vi "exo4.vi"() -> ()   [LabVIEW 2019]
uses:
  <vilib>/myRIO/Instrument Drivers/Onboard IO/I2C/typedefs/I2C User Configuration.ctl
  <vilib>/myRIO/Instrument Drivers/Onboard IO/I2C/typedefs/I2C Transfer Rate.ctl
  <vilib>/myRIO/Instrument Drivers/Onboard IO/I2C/typedefs/I2C Reference.ctl
  <vilib>/myRIO/Common/Instrument Driver Framework/Utilities/typedefs/myRIO Generic Hardware Reference.ctl
  <vilib>/myRIO/Common/Instrument Driver Framework/Utilities/typedefs/Hardware Version Enum.ctl
  <vilib>/myRIO/Common/Instrument Driver Framework/Utilities/typedefs/myRIO v1.0 Reference.ctl
  <vilib>/myRIO/Common/Instrument Driver Framework/Utilities/typedefs/Generic FPGA Reference.ctl
  <vilib>/myRIO/Common/Instrument Driver Framework/myRIO v1.0/I2C/typedefs/I2C Channels Enum.ctl
  <vilib>/myRIO/Instrument Drivers/Onboard IO/I2C/typedefs/I2C Configuration.ctl
  <vilib>/userDefined/High Color/nirio_resource_hc.ctl
  <vilib>/myRIO/Common/Instrument Driver Framework/Utilities/vis/Is FPGA Ref Available.vi
  <vilib>/myRIO/Common/Instrument Driver Framework/myRIO v1.0/I2C/vis/myRIO v1.1 Open I2C.vi
  <vilib>/myRIO/Instrument Drivers/Onboard IO/I2C/vis/Configure.vi
  <vilib>/myRIO/Instrument Drivers/Onboard IO/I2C/vis/Write.vi
  <vilib>/myRIO/Instrument Drivers/Onboard IO/I2C/vis/Read.vi
  <vilib>/myRIO/Common/Instrument Driver Framework/Utilities/vis/Validate Channels.vi
  <vilib>/myRIO/Common/Instrument Driver Framework/myRIO v1.0/I2C/vis/myRIO v1.0 Reserve I2C.vi
  <vilib>/myRIO/Common/Instrument Driver Framework/myRIO v1.0/I2C/vis/myRIO v1.0 Build MUX Configuration I2C.vi
  <vilib>/myRIO/Common/Instrument Driver Framework/myRIO v1.0/Resource Manager/vis/myRIO v1.0 Reserve Channel List.vi
  <vilib>/myRIO/Common/Instrument Driver Framework/myRIO v1.0/Resource Manager/vis/myRIO v1.0 Create Configuration List.vi
  <vilib>/myRIO/Common/Instrument Driver Framework/myRIO v1.0/Resource Manager/vis/myRIO v1.0 Reserve Channel.vi
  <vilib>/myRIO/Common/Instrument Driver Framework/myRIO v1.0/Resource Manager/vis/myRIO v1.0 Unreserve Channel.vi
  <vilib>/myRIO/Common/Instrument Driver Framework/myRIO v1.0/Resource Manager/vis/myRIO v1.0 Build Mutex Name.vi
  <vilib>/Utility/VariantDataType/GetNumericInfo.vi
  <vilib>/Utility/error.llb/Error Cluster From Error Code.vi
  <vilib>/myRIO/Common/Instrument Driver Framework/myRIO v1.0/myRIO v1.1 Open.vi
  <vilib>/myRIO/Common/Instrument Driver Framework/Utilities/vis/IO Manager.vi
  <vilib>/myRIO/Common/Instrument Driver Framework/Utilities/vis/Configuration Manager.vi
  <vilib>/myRIO/Common/Instrument Driver Framework/myRIO v1.0/Resource Manager/vis/myRIO v1.0 Configure IO.vi
  <vilib>/myRIO/Common/Instrument Driver Framework/myRIO v1.0/myRIO v1.0 Close.vi
  <vilib>/myRIO/Common/Instrument Driver Framework/myRIO v1.0/I2C/vis/myRIO v1.0 Configure I2C.vi
  <vilib>/myRIO/Common/Instrument Driver Framework/myRIO v1.0/I2C/vis/myRIO v1.0 Write I2C.vi
  <vilib>/myRIO/Common/Instrument Driver Framework/myRIO v1.0/I2C/vis/myRIO v1.0 Read I2C.vi
  <vilib>/myRIO/Express VI/Onboard IO/I2C/I2C Express VI.xnode
  <vilib>/myRIO/Instrument Drivers/Onboard IO/I2C/vis/myRIO I2C Open.xnode
  <vilib>/myRIO/Instrument Drivers/Onboard IO/I2C/I2C.lvlib
panel:
  out "Bytes Read Z high magnetometer":u8[](array[numeric])
  out "Bytes Read Y high magnetometer":u8[](array[numeric])
  out "Bytes Read X high magnetometer":u8[](array[numeric])
  out "Bytes Bytes Read Z low magnetometer":u8[](array[numeric])
  out "Bytes Bytes Read Y low magnetometer":u8[](array[numeric])
  out "Bytes Bytes Read X low magnetometer":u8[](array[numeric])
  out "Bytes Read Z high accelerometer":u8[](array[numeric])
  out "Bytes Read Y high accelerometer":u8[](array[numeric])
  out "Bytes Read X high accelerometer":u8[](array[numeric])
  out "Bytes Read Z low accelerometer":u8[](array[numeric])
  out "Bytes Read Y low accelerometer":u8[](array[numeric])
  out "Bytes Read X low accelerometer":u8[](array[numeric])
  in  "stop":bool
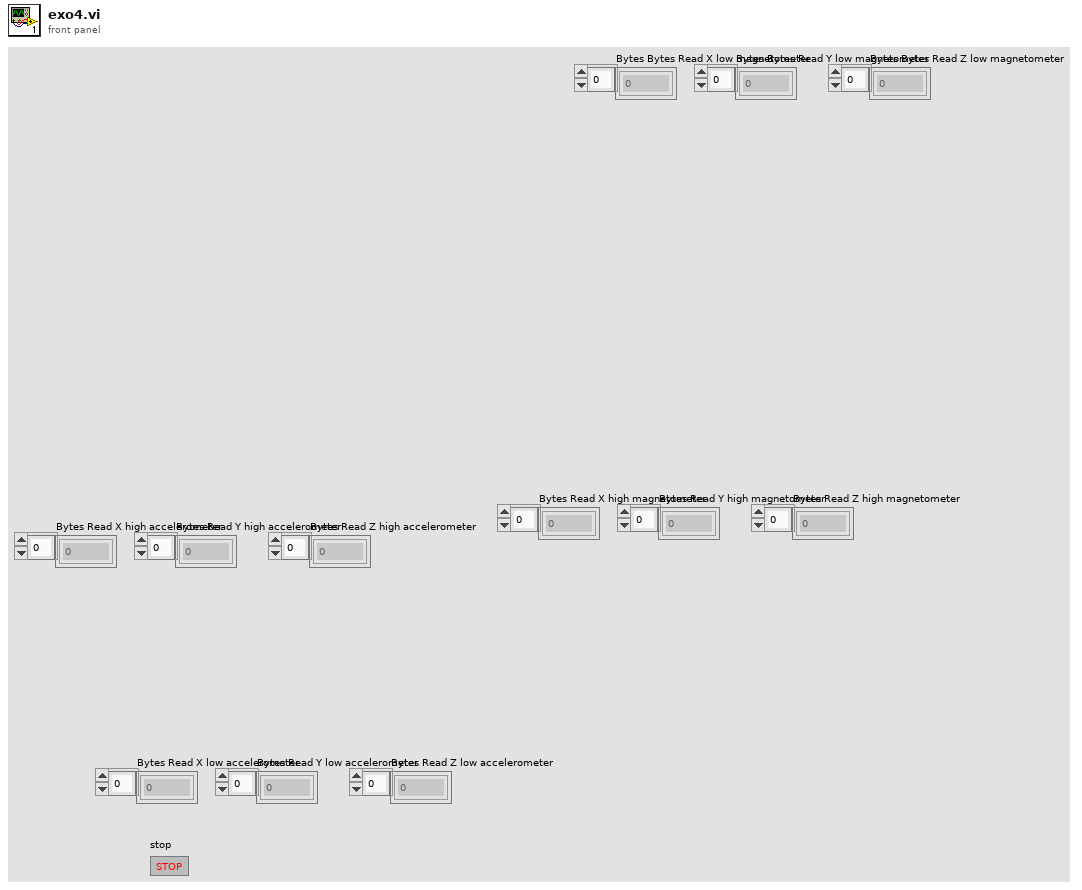
[diagram p1: front panel]
types:
  T1 = enum16{"open", "replace", "create", "open or create", "replace or create", "replace or create with confirmation"}
  T2 = typedef "I2C.lvlib/I2C Reference.ctl" = cluster{"myRIO Reference":T3, "I2C Channels Enum":T7, "I2C Configuration":T8}
  T3 = typedef "myRIO Generic Hardware Reference.ctl" = cluster{"myRIO Model":T4, "myRIO Hardware Reference":T5}
  T4 = typedef "Hardware Version Enum.ctl" = enum16{"Unknown", "myRIO-1900", "myRIO-1950", "roboRIO", "NI ELVIS RIO CM", "ELVIS III"}
  T5 = typedef "myRIO v1.0 Reference.ctl" = cluster{"Generic FPGA Reference":T6, "Allow multiple opens":bool}
  T6 = typedef "Generic FPGA Reference.ctl" = refnum<k20>
  T7 = typedef "I2C Channels Enum.ctl" = enum16{"Not Connected", "A/I2C", "B/I2C", "I2C/I2C"}
  T8 = typedef "I2C.lvlib/I2C Configuration.ctl" = cluster{"I2C Transfer Rate":T9}
  T9 = typedef "I2C.lvlib/I2C Transfer Rate.ctl" = enum16{"Standard mode (100 kbps)", "Fast mode (400 kbps)"}
  T10 = typedef "I2C.lvlib/I2C User Configuration.ctl" = cluster{"I2C Transfer Rate":T9}
  T11 = typedef "nirio_resource_hc.ctl" = tag
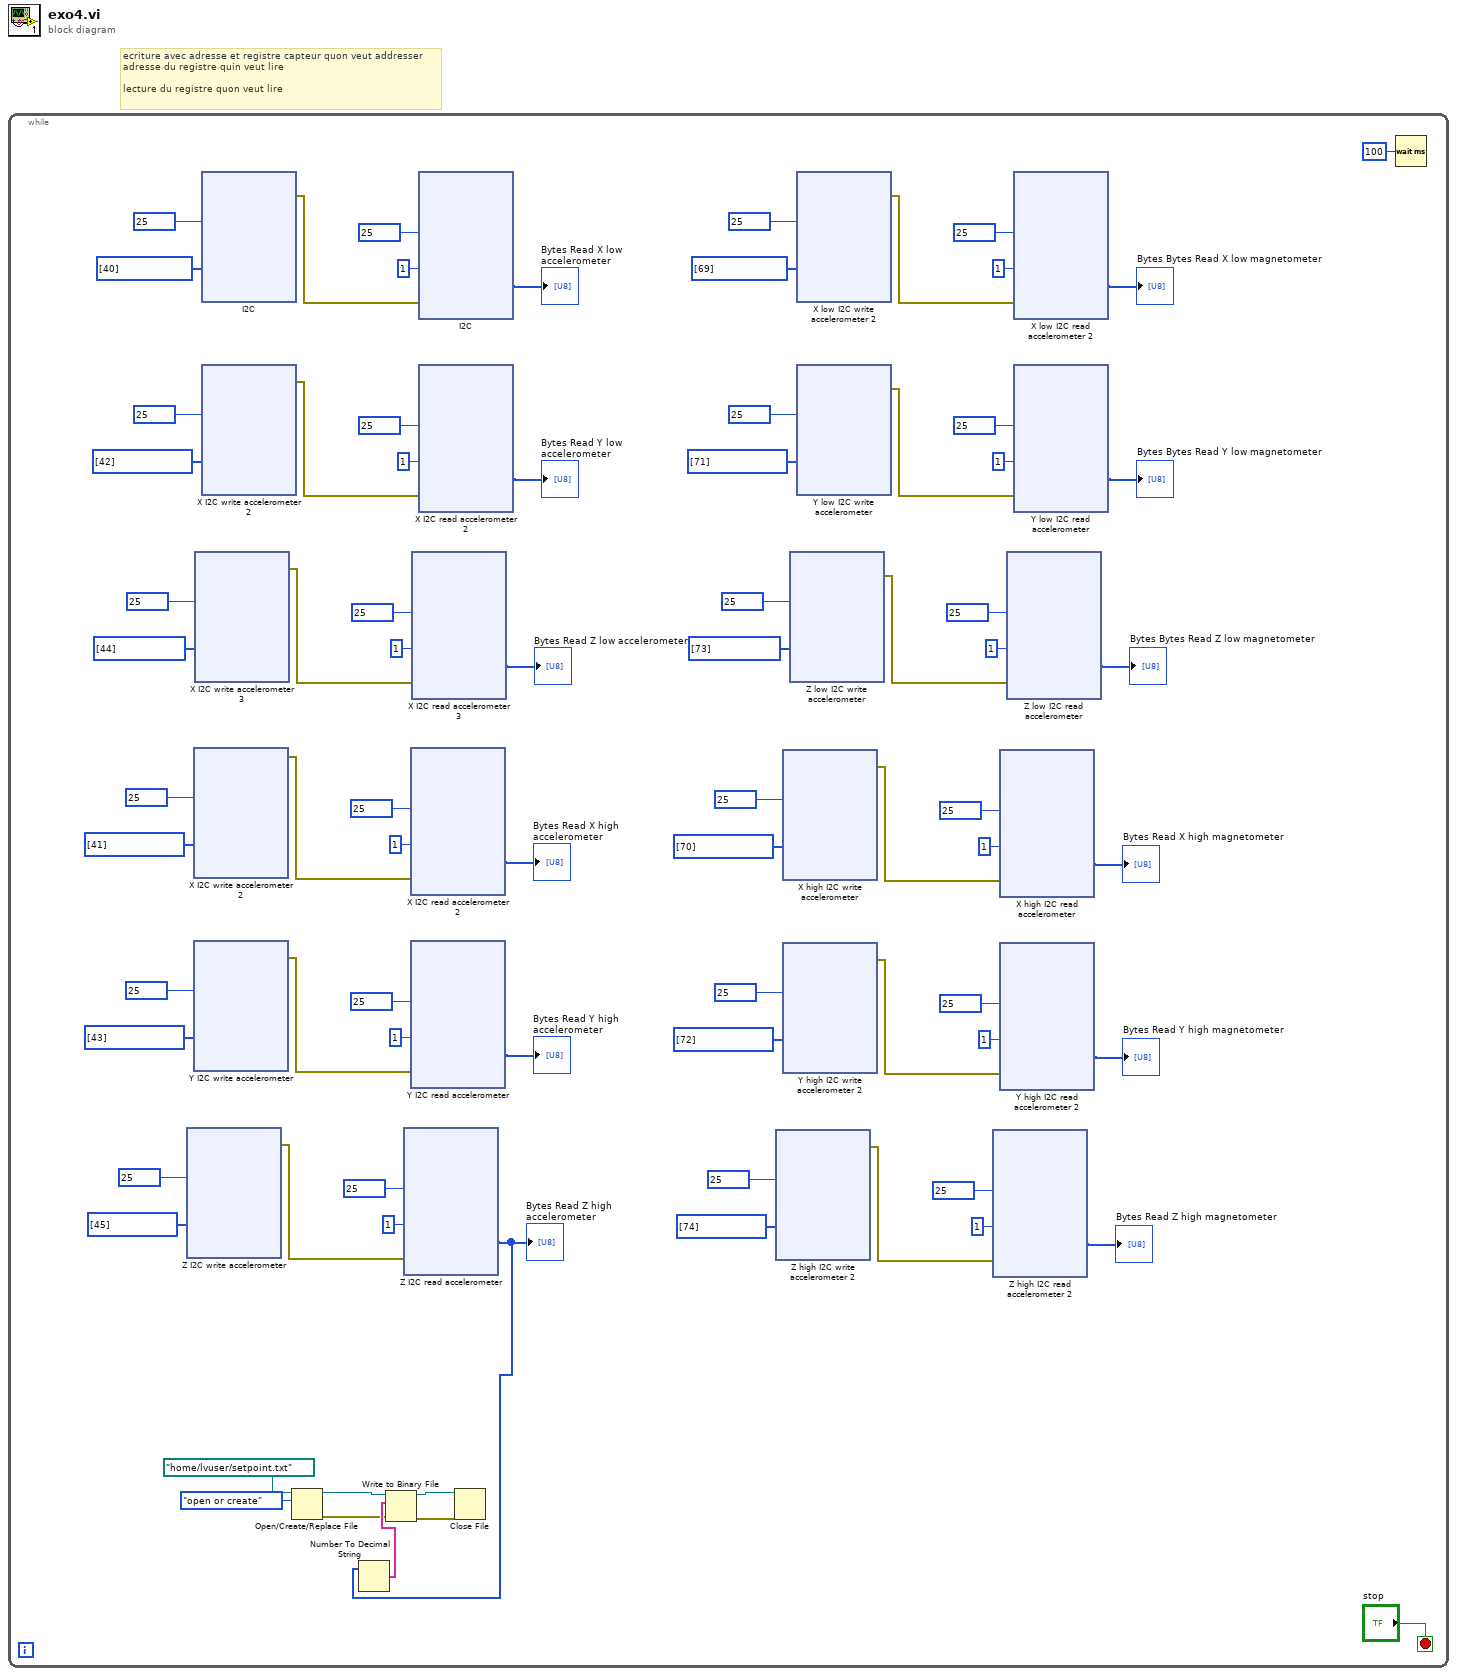
[diagram p0: block diagram]
diagram:
  # "ecriture avec adresse et registre capteur quon veut addresser\nadresse du registre quin veut lire\n\nlecture du registre quon veut lire"
  n1 = while {
    stop <- "stop" stop-if-true
    n2 = xnode "Z I2C write accelerometer"("Slave Address (7-bit)"=u8 25, "Bytes to Write"=u8[] [45]) -> ("error out"=w54:errorcluster)  [unwired: 1 in]
    n3 = xnode "X I2C write accelerometer 2"("Slave Address (7-bit)"=u8 25, "Bytes to Write"=u8[] [41]) -> ("error out"=w64:errorcluster)  [unwired: 1 in]
    n4 = xnode "Y I2C write accelerometer"("Slave Address (7-bit)"=u8 25, "Bytes to Write"=u8[] [43]) -> ("error out"=w59:errorcluster)  [unwired: 1 in]
    n5 = xnode "X I2C write accelerometer 3"("Slave Address (7-bit)"=u8 25, "Bytes to Write"=u8[] [44]) -> ("error out"=w69:errorcluster)  [unwired: 1 in]
    n6 = xnode "I2C"("Slave Address (7-bit)"=u8 25, "Bytes to Write"=u8[] [40]) -> ("error out"=w79:errorcluster)  [unwired: 1 in]
    n7 = xnode "X I2C write accelerometer 2"("Slave Address (7-bit)"=u8 25, "Bytes to Write"=u8[] [42]) -> ("error out"=w74:errorcluster)  [unwired: 1 in]
    n8 = Open/Create/Replace File(file path (use dialog)=path "/home/lvuser/setpoint.txt", operation (0:open)=T1."open or create") -> (refnum out=w43:refnum<file>, error out=w41:errorcluster)  [unwired: 4 in, 1 out]
    n9 = xnode "Z I2C read accelerometer"("Slave Address (7-bit)"=u8 25, "Byte Count"=u32 1, "error in (no error)"=w54) -> ("Bytes Read"=w37:u8[])  [unwired: 1 out]
    "Bytes Read Z high accelerometer" <- w37
    n10 = Number To Decimal String(number=w37) -> (decimal integer string=w42:string[])  [unwired: 1 in]
    n11 = Write to Binary File(file (use dialog)=w43, data=w42, error in=w41) -> (refnum out=w40:refnum<file>, error out=w39:errorcluster)  [unwired: 3 in, 1 out]
    n12 = xnode "X I2C read accelerometer 2"("Slave Address (7-bit)"=u8 25, "Byte Count"=u32 1, "error in (no error)"=w64) -> ("Bytes Read"=→"Bytes Read X high accelerometer":u8[])  [unwired: 1 out]
    n13 = xnode "Y I2C read accelerometer"("Slave Address (7-bit)"=u8 25, "Byte Count"=u32 1, "error in (no error)"=w59) -> ("Bytes Read"=→"Bytes Read Y high accelerometer":u8[])  [unwired: 1 out]
    n14 = xnode "X I2C read accelerometer 3"("Slave Address (7-bit)"=u8 25, "Byte Count"=u32 1, "error in (no error)"=w69) -> ("Bytes Read"=→"Bytes Read Z low accelerometer":u8[])  [unwired: 1 out]
    n15 = xnode "I2C"("Slave Address (7-bit)"=u8 25, "Byte Count"=u32 1, "error in (no error)"=w79) -> ("Bytes Read"=→"Bytes Read X low accelerometer":u8[])  [unwired: 1 out]
    n16 = xnode "X I2C read accelerometer 2"("Slave Address (7-bit)"=u8 25, "Byte Count"=u32 1, "error in (no error)"=w74) -> ("Bytes Read"=→"Bytes Read Y low accelerometer":u8[])  [unwired: 1 out]
    n17 = Close File(refnum=w40, error in=w39) -> ()  [unwired: 2 out]
    n18 = xnode "Z high I2C write accelerometer 2"("Slave Address (7-bit)"=u8 25, "Bytes to Write"=u8[] [74]) -> ("error out"=w8:errorcluster)  [unwired: 1 in]
    n19 = xnode "X high I2C write accelerometer"("Slave Address (7-bit)"=u8 25, "Bytes to Write"=u8[] [70]) -> ("error out"=w18:errorcluster)  [unwired: 1 in]
    n20 = xnode "Y high I2C write accelerometer 2"("Slave Address (7-bit)"=u8 25, "Bytes to Write"=u8[] [72]) -> ("error out"=w13:errorcluster)  [unwired: 1 in]
    n21 = xnode "Z low I2C write accelerometer"("Slave Address (7-bit)"=u8 25, "Bytes to Write"=u8[] [73]) -> ("error out"=w26:errorcluster)  [unwired: 1 in]
    n22 = xnode "X low I2C write accelerometer 2"("Slave Address (7-bit)"=u8 25, "Bytes to Write"=u8[] [69]) -> ("error out"=w36:errorcluster)  [unwired: 1 in]
    n23 = xnode "Y low I2C write accelerometer"("Slave Address (7-bit)"=u8 25, "Bytes to Write"=u8[] [71]) -> ("error out"=w31:errorcluster)  [unwired: 1 in]
    n24 = xnode "Z high I2C read accelerometer 2"("Slave Address (7-bit)"=u8 25, "Byte Count"=u32 1, "error in (no error)"=w8) -> ("Bytes Read"=→"Bytes Read Z high magnetometer":u8[])  [unwired: 1 out]
    n25 = xnode "X high I2C read accelerometer"("Slave Address (7-bit)"=u8 25, "Byte Count"=u32 1, "error in (no error)"=w18) -> ("Bytes Read"=→"Bytes Read X high magnetometer":u8[])  [unwired: 1 out]
    n26 = xnode "Y high I2C read accelerometer 2"("Slave Address (7-bit)"=u8 25, "Byte Count"=u32 1, "error in (no error)"=w13) -> ("Bytes Read"=→"Bytes Read Y high magnetometer":u8[])  [unwired: 1 out]
    n27 = xnode "Z low I2C read accelerometer"("Slave Address (7-bit)"=u8 25, "Byte Count"=u32 1, "error in (no error)"=w26) -> ("Bytes Read"=→"Bytes Bytes Read Z low magnetometer":u8[])  [unwired: 1 out]
    n28 = xnode "X low I2C read accelerometer 2"("Slave Address (7-bit)"=u8 25, "Byte Count"=u32 1, "error in (no error)"=w36) -> ("Bytes Read"=→"Bytes Bytes Read X low magnetometer":u8[])  [unwired: 1 out]
    n29 = xnode "Y low I2C read accelerometer"("Slave Address (7-bit)"=u8 25, "Byte Count"=u32 1, "error in (no error)"=w31) -> ("Bytes Read"=→"Bytes Bytes Read Y low magnetometer":u8[])  [unwired: 1 out]
    n30 = Wait (ms)(milliseconds to wait=u32 100) -> ()  [unwired: 1 out]
  }
